vi "Config Drive Pipeline Command.vi"(8 "Command Info In":T2, 10 "Drive Conditions":T1={"Field Centric"=TRUE, "Auto Corretion"=FALSE, "Theta Align"=FALSE}) -> (0 "Command Info Out":T2)   [LabVIEW 2025]
uses:
  Framework/Robot Global Data.vi
  <vilib>/Rock Robotics/WPI/Framework/Completion Status.ctl
  <vilib>/Rock Robotics/WPI/Framework/Completion Notifier.ctl
  <vilib>/Rock Robotics/WPI/Framework/Command Status Info.ctl
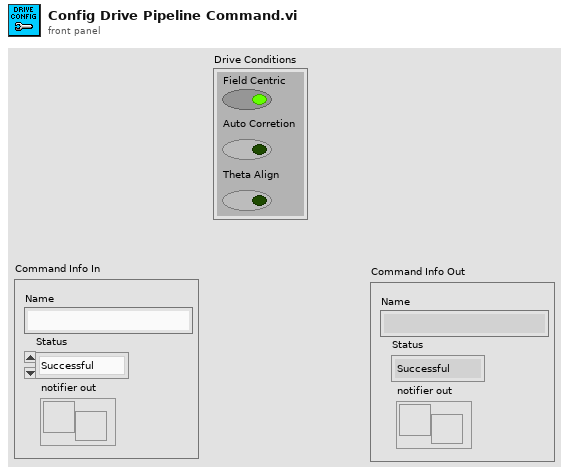
[diagram p1: front panel]
types:
  T1 = cluster{"Field Centric":bool, "Auto Corretion":bool, "Theta Align":bool}
  T2 = typedef "Command Status Info.ctl" = cluster{"Name":string, "Status":T3, "notifier out":T4}
  T3 = typedef "Completion Status.ctl" = enum16{"Successful", "Aborted", "Incomplete"}
  T4 = typedef "Completion Notifier.ctl" = refnum<notifier>
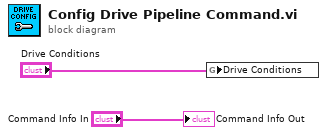
[diagram p0: block diagram]
diagram:
  n1 = global write "Robot Global Data.vi" "Drive Conditions"("Drive Conditions") -> ()
  "Command Info Out" <- "Command Info In"
